vi "ScanSteuerung_RemoveLoops.vi"(0 "ScanSteuerung":T1=[{"Time [s]"=0.0, "action"=enum."Abs", "channel"=enum."SMoveTime", "value (/s)"=0.0008}, {"Time [s]"=0.0, "action"=enum."Abs", "channel"=enum."GalvoX", "value (/s)"=-0.0005000005}, {"Time [s]"=0.0, "action"=enum."Abs", "channel"=enum."GalvoY", "value (/s)"=-0.0005000005}, {"Time [s]"=0.0, "action"=enum."Abs", "channel"=enum."Galvo3", "value (/s)"=0.0}, {"Time [s]"=0.0, "action"=enum."LoopStart", "channel"=enum."Loop", "value (/s)"=10.0}, {"Time [s]"=0.0, "action"=enum."Inc", "channel"=enum."GalvoX", "value (/s)"=0.1000001}, {"Time [s]"=0.0, "action"=enum."Inc", "channel"=enum."GalvoY", "value (/s)"=0.0}, {"Time [s]"=0.0, "action"=enum."Inc", "channel"=enum."Galvo3", "value (/s)"=51200.0}, {"Time [s]"=0.01, "action"=enum."Abs", "channel"=enum."Digital", "value (/s)"=1.0}, {"Time [s]"=0.01, "action"=enum."Inc", "channel"=enum."GalvoX", "value (/s)"=0.0}, {"Time [s]"=0.01, "action"=enum."Inc", "channel"=enum."GalvoY", "value (/s)"=0.625000625}, {"Time [s]"=0.01, "action"=enum."Inc", "channel"=enum."Galvo3", "value (/s)"=0.0}, {"Time [s]"=0.01008, "action"=enum."Abs", "channel"=enum."Digital", "value (/s)"=0.0}, {"Time [s]"=0.01008, "action"=enum."Inc", "channel"=enum."GalvoX", "value (/s)"=-0.1000001}, {"Time [s]"=0.01008, "action"=enum."Inc", "channel"=enum."GalvoY", "value (/s)"=-0.0}, {"Time [s]"=0.01008, "action"=enum."Inc", "channel"=enum."Galvo3", "value (/s)"=-51200.0}, {"Time [s]"=0.02008, "action"=enum."Abs", "channel"=enum."Digital", "value (/s)"=1.0}, {"Time [s]"=0.02008, "action"=enum."Inc", "channel"=enum."GalvoX", "value (/s)"=0.0}, {"Time [s]"=0.02008, "action"=enum."Inc", "channel"=enum."GalvoY", "value (/s)"=0.625000625}, {"Time [s]"=0.02008, "action"=enum."Inc", "channel"=enum."Galvo3", "value (/s)"=0.0}, {"Time [s]"=0.02016, "action"=enum."Abs", "channel"=enum."Digital", "value (/s)"=0.0}, {"Time [s]"=0.02016, "action"=enum."LoopEnd", "channel"=enum."Loop", "value (/s)"=0.0}, {"Time [s]"=0.2016, "action"=enum."Inc", "channel"=enum."GalvoX", "value (/s)"=0.0}, {"Time [s]"=0.2016, "action"=enum."Inc", "channel"=enum."GalvoY", "value (/s)"=0.0}, {"Time [s]"=0.2016, "action"=enum."Inc", "channel"=enum."Galvo3", "value (/s)"=0.0}]) -> (1 "ScanSteuerungOut":T1=[{"Time [s]"=0.0, "action"=enum."Abs", "channel"=enum."SMoveTime", "value (/s)"=0.0008}, {"Time [s]"=0.0, "action"=enum."Abs", "channel"=enum."GalvoX", "value (/s)"=-0.0005000005}, {"Time [s]"=0.0, "action"=enum."Abs", "channel"=enum."GalvoY", "value (/s)"=-0.0005000005}, {"Time [s]"=0.0, "action"=enum."Abs", "channel"=enum."Galvo3", "value (/s)"=0.0}, {"Time [s]"=0.0, "action"=enum."LoopStart", "channel"=enum."Loop", "value (/s)"=10.0}, {"Time [s]"=0.0, "action"=enum."Inc", "channel"=enum."GalvoX", "value (/s)"=1.000001e-06}, {"Time [s]"=0.0, "action"=enum."Inc", "channel"=enum."GalvoY", "value (/s)"=0.0}, {"Time [s]"=0.0, "action"=enum."Inc", "channel"=enum."Galvo3", "value (/s)"=0.512}, {"Time [s]"=999.9999999999999, "action"=enum."Abs", "channel"=enum."Digital", "value (/s)"=1.0}, {"Time [s]"=999.9999999999999, "action"=enum."Inc", "channel"=enum."GalvoX", "value (/s)"=0.0}, {"Time [s]"=999.9999999999999, "action"=enum."Inc", "channel"=enum."GalvoY", "value (/s)"=6.25000625e-06}, {"Time [s]"=999.9999999999999, "action"=enum."Inc", "channel"=enum."Galvo3", "value (/s)"=0.0}, {"Time [s]"=1008.0, "action"=enum."Abs", "channel"=enum."Digital", "value (/s)"=0.0}, {"Time [s]"=1008.0, "action"=enum."Inc", "channel"=enum."GalvoX", "value (/s)"=-1.000001e-06}, {"Time [s]"=1008.0, "action"=enum."Inc", "channel"=enum."GalvoY", "value (/s)"=-0.0}, {"Time [s]"=1008.0, "action"=enum."Inc", "channel"=enum."Galvo3", "value (/s)"=-0.512}, {"Time [s]"=2008.0, "action"=enum."Abs", "channel"=enum."Digital", "value (/s)"=1.0}, {"Time [s]"=2008.0, "action"=enum."Inc", "channel"=enum."GalvoX", "value (/s)"=0.0}, {"Time [s]"=2008.0, "action"=enum."Inc", "channel"=enum."GalvoY", "value (/s)"=6.25000625e-06}, {"Time [s]"=2008.0, "action"=enum."Inc", "channel"=enum."Galvo3", "value (/s)"=0.0}, {"Time [s]"=2016.0, "action"=enum."Abs", "channel"=enum."Digital", "value (/s)"=0.0}, {"Time [s]"=2016.0, "action"=enum."LoopEnd", "channel"=enum."Loop", "value (/s)"=0.0}, {"Time [s]"=20160.0, "action"=enum."Inc", "channel"=enum."GalvoX", "value (/s)"=0.0}, {"Time [s]"=20160.0, "action"=enum."Inc", "channel"=enum."GalvoY", "value (/s)"=0.0}, {"Time [s]"=20160.0, "action"=enum."Inc", "channel"=enum."Galvo3", "value (/s)"=0.0}], 2 "LoopLengths":dbl[](array[numeric]), 3 "Loopelements":i32[](array[numeric]))   [LabVIEW 2011]
uses:
  ScanControl.ctl
  ScanControl_Action.ctl
  ScanControl_Channel.ctl
panel:
  out "subarray":T1
  out "Ends":i32[](array[numeric])
  out "Starts":i32[](array[numeric])
  # "Checked: Scan mit resolveLoops aufgeblasen, und\nhier wieder zusammengeschoben == ist Identisch!\ngeht nicht wenn keine loop da ist!!!"
  # "todo? Add error In and out?"
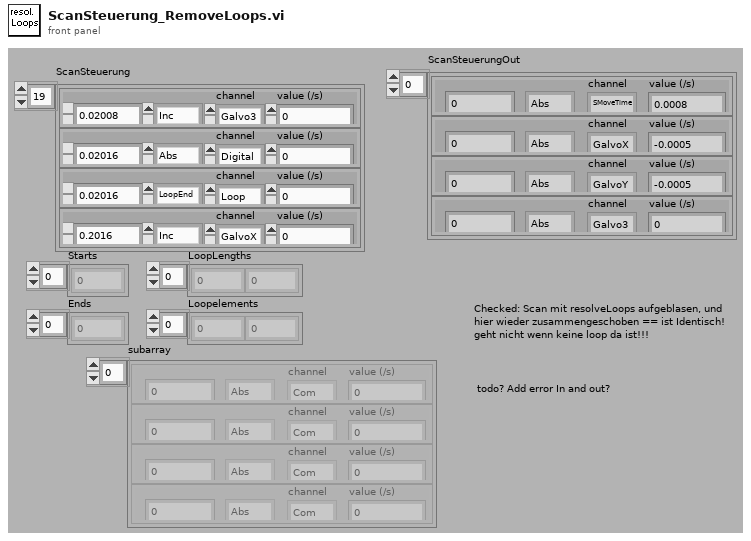
[diagram p1: front panel]
types:
  T1 = typedef "ScanControl.ctl" = cluster{"Time [s]":dbl, "action":T2, "channel":T3, "value (/s)":dbl}[]
  T2 = typedef "ScanControl_Action.ctl" = enum16{"Abs", "Rel", "Inc", "IncInc", "LoopStart", "LoopEnd", "WaitTriggerRising"}
  T3 = typedef "ScanControl_Channel.ctl" = enum16{"Com", "AnalogConfig", "AnalogValue", "GalvoX", "GalvoY", "Galvo3", "Galvo4", "Digital", "Free", "Loop", "SMoveTime", "Image1X", "Image1Y", "Image2X", "Image2Y"}
  T4 = enum16{"Abs", "Rel", "Inc", "IncInc", "LoopStart", "LoopEnd"}
  T5 = cluster{"Zeitpunkt [Basis]":dbl, "Wirkung":enum16{"Abs", "Rel", "Inc", "IncInc", "LoopStart", "LoopEnd"}, "Kanal":enum16{"Com", "Digital", "Analog", "GalvoX", "GalvoY", "GalvoCCD", "Free1", "Free2", "Free3", "Loop", "SMoveTime", "Image1X", "Image1Y", "Image2X", "Image2Y"}, "Wert (/Basis)":dbl}[]
  T6 = cluster{"Time [s]":dbl, "action":T2, "channel":T3, "value (/s)":dbl}
  T7 = cluster{"Time [s]":dbl, "action":T2, "channel":u16, "value (/s)":dbl}[]
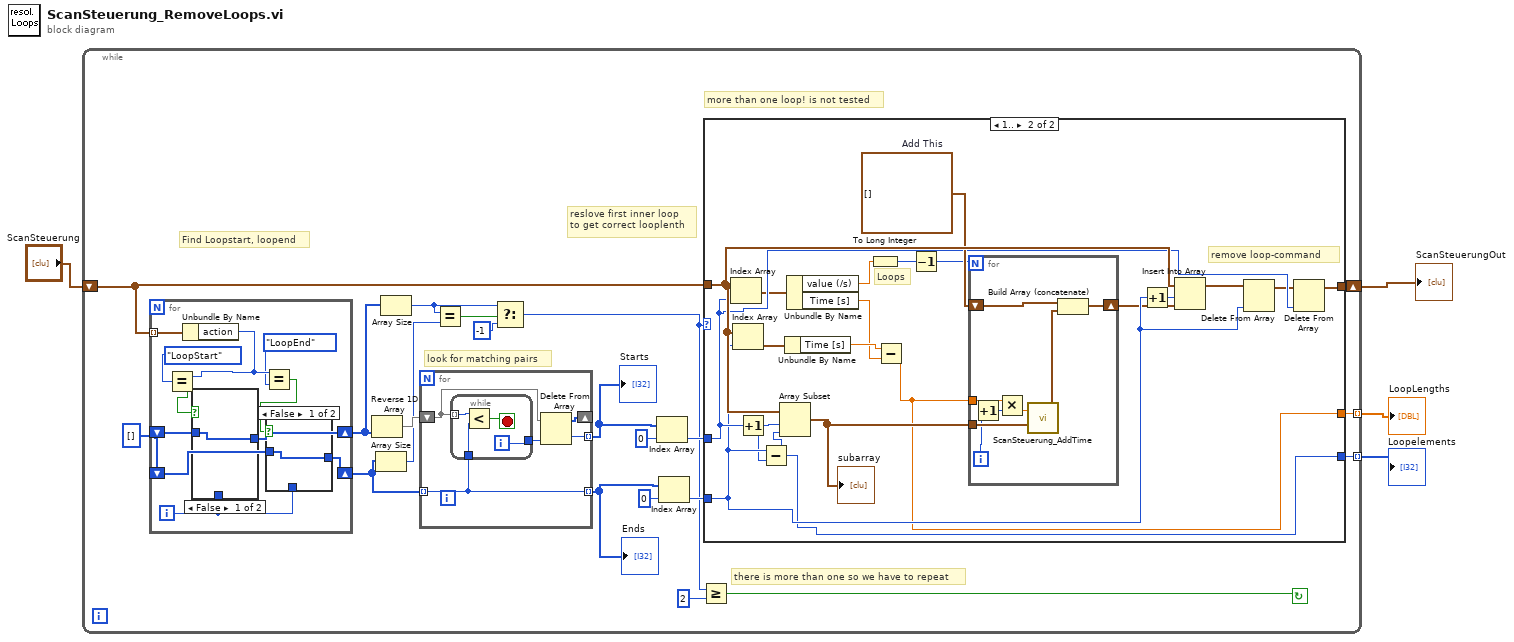
[diagram p0: block diagram]
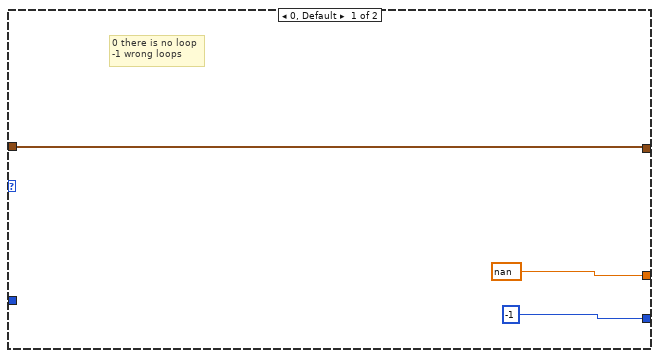
[diagram p2: hidden frame]
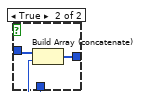
[diagram p3: hidden frame]
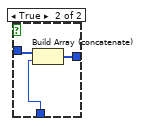
[diagram p4: hidden frame]
diagram:
  n1 = while {
    shift-right: [w19] -> w3
    shift-left: "ScanSteuerung" -> [w24]
    tunnel: [w16] -> w2 mode=indexing
    tunnel: [w15] -> w1 mode=indexing
    stop <- w17 continue-if-true
    w25 = i32[] []
    # "there is more than one so we have to repeat"
    # "reslove first inner loop\nto get correct looplenth"
    # "look for matching pairs"
    # "more than one loop! is not tested"
    # "Find Loopstart, loopend"
    n2 = for {
      tunnel: w24 -> [w76] mode=indexing
      shift-right: [w70] -> w11
      shift-left: w25 -> [w71]
      shift-right: [w67] -> w10
      shift-left: w25 -> [w68]
      i -> [w69]
      n3 = Unbundle By Name(w76) -> ("action"=w75:T2)
      n4 = Equal?(x=w75, y=T4."LoopStart" ("Wirkung")) -> (x = y?=w72:bool)
      n5 = case shown="False" w72 {
        tunnel: w71 -> [w81 w83]
        tunnel: w69 -> [_ w84]
        tunnel: [w81 w82] -> w70
        frame False {
        }
        frame True {
          n6 = Build Array (concatenate)(w83, w84) -> (w82:i32[])
        }
      }
      n7 = Equal?(x=w75, y=T4."LoopEnd" ("Wirkung")) -> (x = y?=w66:bool)
      n8 = case shown="False" w66 {
        tunnel: w68 -> [w77 w79]
        tunnel: w69 -> [_ w80]
        tunnel: [w77 w78] -> w67
        frame False {
        }
        frame True {
          n9 = Build Array (concatenate)(w79, w80) -> (w78:i32[])
        }
      }
    }
    n10 = Reverse 1D Array(array=w11) -> (reversed array=w14:i32[])
    n11 = Array Size(array=w10) -> (size(s)=w9:i32)
    n12 = Array Size(array=w11) -> (size(s)=w8:i32)
    n13 = for {
      tunnel: w10 -> [w27] mode=indexing
      tunnel: [w28] -> w12 mode=indexing
      tunnel: [w27] -> w13 mode=indexing
      shift-right: [w26] -> _
      shift-left: w14 -> [w30]
      n14 = while {
        tunnel: w30 -> [w31] mode=indexing
        tunnel: w27 -> [w34]
        tunnel: [w33] -> w29
        i -> [w33]
        stop <- w32 stop-if-true
        n15 = Less?(x=w31, y=w34) -> (x < y?=w32:bool)
      }
      n16 = Delete From Array(array=w30, index=w29) -> (deleted portion=w28:i32, array with subset deleted=w26:i32[])  [unwired: 1 in]
    }
    "Starts" <- w12
    "Ends" <- w13
    n17 = Equal?(x=w8, y=w9) -> (x = y?=w6:bool)
    n18 = Select(t=w8, s=w6, f=-1) -> (s? t:f=w7:i32)
    n19 = Index Array(array=w12, index=0) -> (element=w22:i32)
    n20 = Index Array(array=w13, index=0) -> (element=w21:i32)
    n21 = Greater Or Equal?(x=w7, y=2) -> (x >= y?=w17:bool)
    n22 = case shown="1.." w7 {
      tunnel: w24 -> [w37 w57]
      tunnel: w22 -> [_ w55]
      tunnel: w21 -> [_ w54]
      tunnel: [w37 w40] -> w19
      tunnel: [nan w39] -> w16
      tunnel: [-1 w38] -> w15
      frame 0, Default {
        # "0 there is no loop\n-1 wrong loops"
      }
      frame 1.. {
        w56 = T5 []  # Add This
        # "remove loop-command"
        # "Loops"
        n23 = Index Array(array=w57, index=w55) -> (element=w53:T6)
        n24 = Index Array(array=w57, index=w54) -> (element=w52:T6)
        n25 = Increment(x=w55) -> (x+1=w49:i32)
        n26 = Subtract(x=w54, y=w49) -> (x-y=w38:i32)
        n27 = Array Subset(array=w57, index=w49, length=w38) -> (w46:T1)
        "subarray" <- w46
        n28 = Unbundle By Name(w52) -> ("Time [s]"=w51:dbl)
        n29 = Unbundle By Name(w53) -> ("value (/s)"=w48:dbl, "Time [s]"=w50:dbl)
        n30 = To Long Integer(number=w48) -> (32bit integer=w47:i32)
        n31 = Subtract(x=w51, y=w50) -> (x-y=w39:dbl)
        n32 = Decrement(x=w47) -> (x-1=w41:i32)
        n33 = for {
          N: w41 -> [_]
          tunnel: w46 -> [w65]
          tunnel: w39 -> [w62]
          shift-right: [w59] -> w45
          shift-left: w56 -> [w61]
          i -> [w63]
          n34 = Increment(x=w63) -> (x+1=w58:i32)
          n35 = Multiply(x=w62, y=w58) -> (x*y=w64:dbl)
          n36 = call "ScanSteuerung_AddTime.vi"("ScanSteuerung"=w65, "Add Time"=w64) -> ("ScanSteuerungOut"=w60:T1)
          n37 = Build Array (concatenate)(w61, w60) -> (w59:T7)
        }
        n38 = Increment(x=w54) -> (x+1=w44:i32)
        n39 = Insert Into Array(array=w57, index=w44, new element=w45) -> (w43:T1)
        n40 = Delete From Array(array=w43, index=w54) -> (array with subset deleted=w42:T1)  [unwired: 1 in, 1 out]
        n41 = Delete From Array(array=w42, index=w55) -> (array with subset deleted=w40:T1)  [unwired: 1 in, 1 out]
      }
    }
  }
  "ScanSteuerungOut" <- w3
  "LoopLengths" <- w2
  "Loopelements" <- w1
